vi "Read Cursor Position.vi"(8 "error in (no error)":errorcluster, 11 "VISA resource name":refnum<visa-resource-name>) -> (0 "error out":errorcluster, 2 "Cursor Position":T1, 3 "VISA resource name out":refnum<visa-resource-name>)   [LabVIEW 2013, in "SRS SR400.lvlib"]
doc: "<B>SC</B>\n\nThe SC command reads the cursor position. \"0\" is returned for left, \"1\" for right, and \"2\" for inactive. To move the cursor, use the CK command."
uses:
  <instrlib>/SRS SR400/SRS SR400.lvlib
  <instrlib>/SRS SR400/Public/Typedefs/Cursor Position.ctl
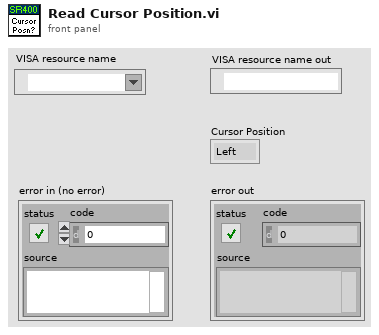
[diagram p1: front panel]
types:
  T1 = typedef "SRS SR400.lvlib/Cursor Position.ctl" = enum16{"Left", "Right", "Inactive"}
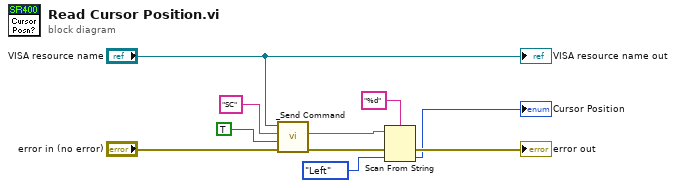
[diagram p0: block diagram]
diagram:
  n1 = call <instrlib>:"_Send Command.vi"("error in (no error)"="error in (no error)", "Read Value? (F)"=TRUE, "Command"="SC" ("command"), "VISA resource name"="VISA resource name") -> ("error out"=w7:errorcluster, "Response"=w8:string)  [unwired: 6 out]
  n2 = Scan From String(format string="%d", input string=w8, error in=w7, default 1=Cursor_Position."Left" ("default value 1")) -> (error out=→"error out":errorcluster, output 1=→"Cursor Position":T1)  [unwired: 1 in, 2 out]
  "VISA resource name out" <- "VISA resource name"
